vi "Read Build Time Output Directory.vi"(8 "error in (no error)":errorcluster, 11 "NSIS Installer in":refnum<class "NSIS Installer.lvclass">) -> (0 "error out":errorcluster, 2 "Build Time Output Directory":path, 3 "NSIS Installer out":refnum<class "NSIS Installer.lvclass">)   [LabVIEW 2017, in "CL_G3_VIComponentBuilder.lvlib" / "NSIS Installer.lvclass"]
uses:
  NSIS Installer.lvclass
  NSIS Installer.lvclass/NSIS Installer.ctl
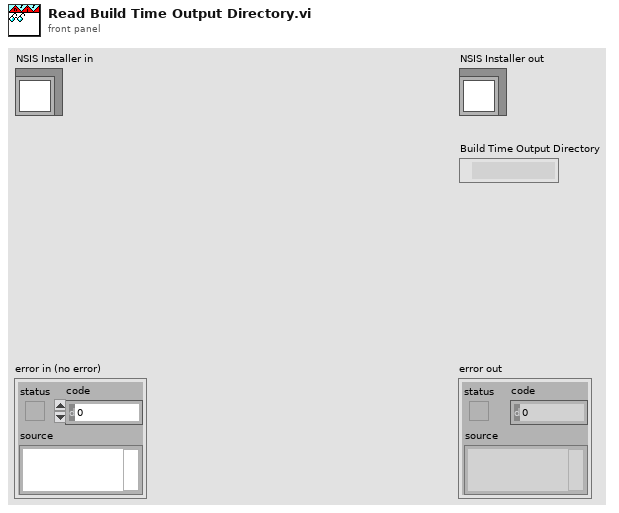
[diagram p1: front panel]
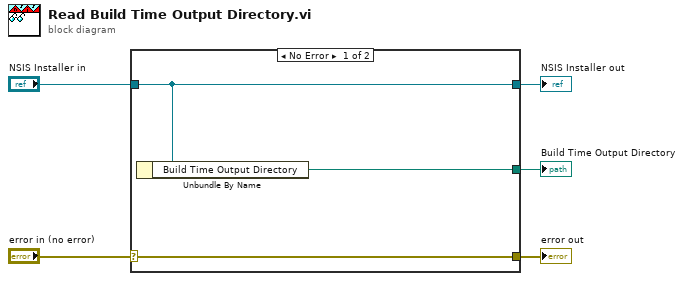
[diagram p0: block diagram]
diagram:
  n1 = case shown="No Error" "error in (no error)" {
    selector: "error in (no error)" -> [w8 w9]
    tunnel: [w8 w9] -> w4
    tunnel: [w7 w10] -> w2
    tunnel: "NSIS Installer in" -> [w7 w10]
    tunnel: [w6 _] -> w1
    frame No Error {
      n2 = Unbundle By Name(w7) -> ("Build Time Output Directory"=w6:path)
    }
    frame Error {
    }
  }
  "error out" <- w4
  "NSIS Installer out" <- w2
  "Build Time Output Directory" <- w1
